vi "Server Loops.vi"(11 "TCPMessaging in":refnum<class "TCPMessaging.lvclass">) -> ()   [LabVIEW 2020, in "Vecto.lvlib" / "TCPMessaging.lvclass"]
uses:
  TCPMessaging.lvclass
  TCPMessaging.lvclass/TCPMessaging.ctl
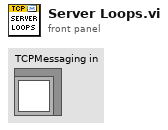
[diagram p1: front panel]
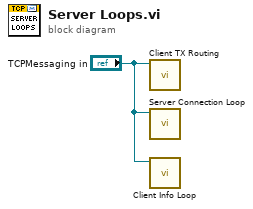
[diagram p0: block diagram]
diagram:
  n1 = call "Client TX Routing.vi"("TCPMessaging in"="TCPMessaging in") -> ()  [unwired: 10 in, 1 out]
  n2 = call "Server Connection Loop.vi"("TCPMessaging in"="TCPMessaging in") -> ()  [unwired: 10 in, 1 out]
  n3 = call "Client Info Loop.vi"("TCPMessaging in"="TCPMessaging in") -> ()  [unwired: 10 in, 1 out]
